vi "Close.vi"(8 "error in (no error)":errorcluster, 11 "NHRDCModel in":refnum<class "NHRDCPowerModel.lvclass">) -> (0 "error out":errorcluster, 3 "NHRDCModel out":refnum<class "NHRDCPowerModel.lvclass">)   [LabVIEW 2018, in "AcPwrPlugins.lvlib" / "NHRDCPowerModel.lvclass"]
doc: "This VI closes the reference to the instrument(s)."
uses:
  NHRDCPowerModel.lvclass
  NHRDCPowerModel.lvclass/NHRDCPowerModel.ctl
  Database/DatabaseBaseClass/DatabaseBaseClass.lvclass
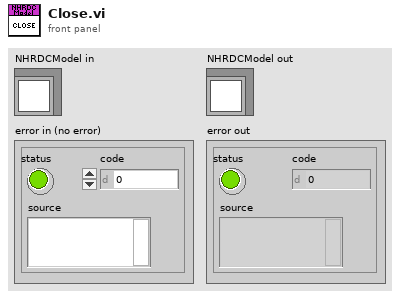
[diagram p1: front panel]
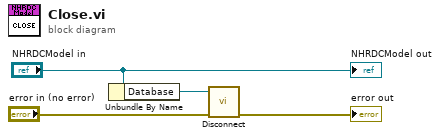
[diagram p0: block diagram]
diagram:
  n1 = Unbundle By Name("NHRDCModel in") -> ("Database"=w3:refnum<class "DatabaseBaseClass.lvclass">)
  n2 = call-dynamic "Disconnect.vi"("error in (no error)"="error in (no error)", "DatabaseBaseClass in"=w3) -> ("error out"=→"error out":errorcluster)  [unwired: 8 in, 1 out]
  "NHRDCModel out" <- "NHRDCModel in"
